vi "Fixed Number Graph Read.vi"(8 "error in":errorcluster, 9 "Data to read in":T2, 10 "Channel_Timing in":T1, 11 "Report Viewer in":refnum<class "Report Viewer.lvclass">) -> (0 "error out":errorcluster, 1 "Data to read out":T2, 2 "Channel_Timing out":T1, 3 "Report Viewer out":refnum<class "Report Viewer.lvclass">, 4 "Waveform":waveform(dbl))   [LabVIEW 2019, in "Report Viewer.lvlib" / "Report Viewer.lvclass"]
uses:
  Library/Report Viewer.lvclass
  Custom Controls/Channel_Timing.ctl
  Custom Controls/Data to Read.ctl
  Library/Report Viewer.lvclass/Report Viewer.ctl
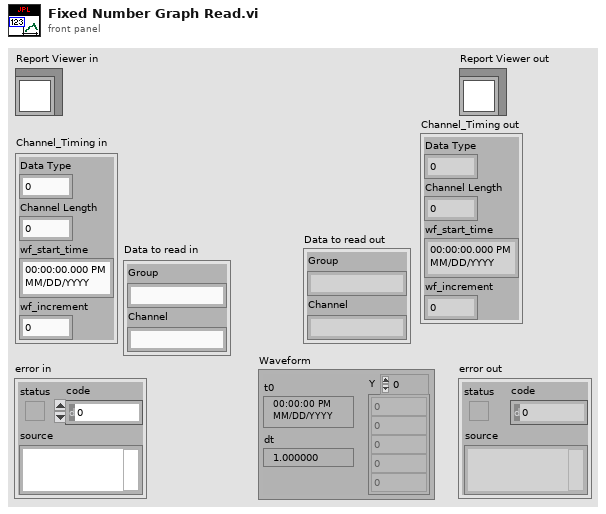
[diagram p1: front panel]
types:
  T1 = typedef "Report Viewer.lvlib/Report Viewer.lvclass/Channel_Timing.ctl" = cluster{"Data Type":u16, "Channel Length":u64, "wf_start_time":timestamp, "wf_increment":dbl}
  T2 = typedef "Report Viewer.lvlib/Report Viewer.lvclass/Data to Read.ctl" = cluster{"Group":string, "Channel":string}
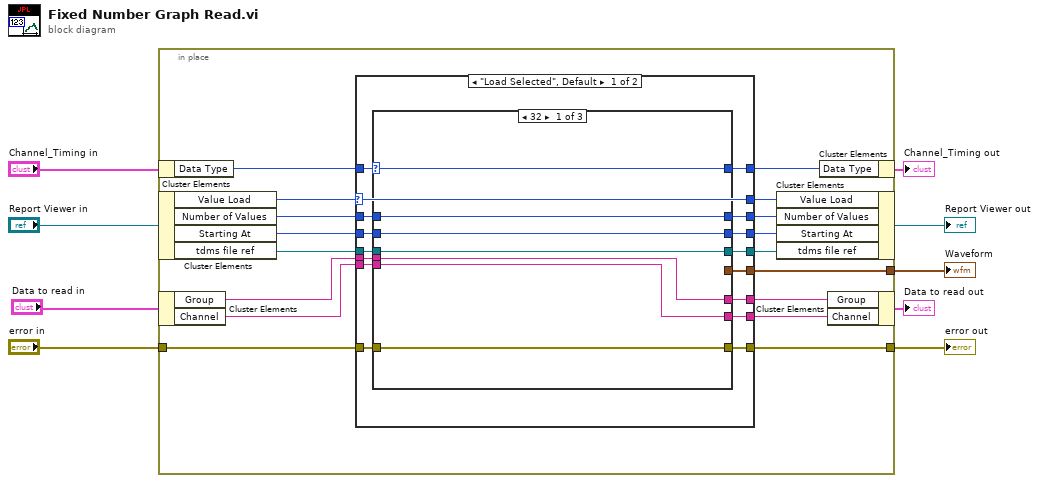
[diagram p0: block diagram]
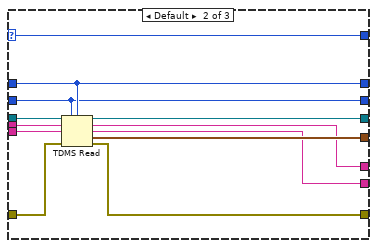
[diagram p2: hidden frame]
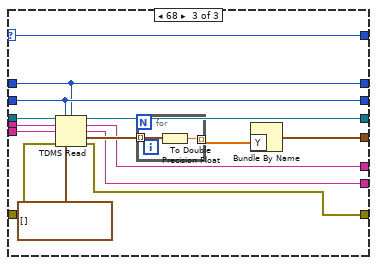
[diagram p3: hidden frame]
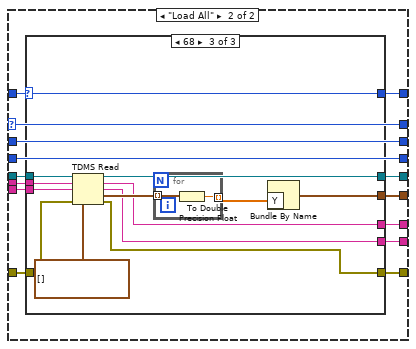
[diagram p4: hidden frame]
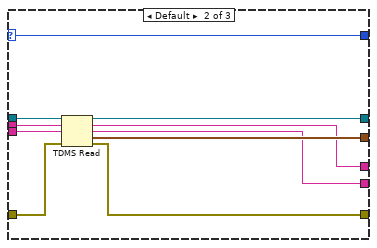
[diagram p6: hidden frame]
diagram:
  n1 = in-place {
    in-place-border: [w24] -> w7
    in-place-border: "error in" -> [w23]
    in-place-border: [w18] -> w3
    n2 = in-place-cluster #1("Channel_Timing in") -> ("Data Type"=w20:u16)
    n3 = in-place-cluster #2("Report Viewer in") -> ("Value Load"=w11:enum32{"Load All", "Load Selected"}, "Number of Values"=w21:i32, "Starting At"=w22:i32, "tdms file ref"=w26:refnum<k34>)
    n4 = in-place-cluster #3("Data to read in") -> ("Group"=w15:string, "Channel"=w14:string)
    n5 = case shown="\"Load Selected\", Default" w11 {
      selector: w11 -> [w27 w79]
      tunnel: w26 -> [w42 w92]
      tunnel: [w41 w91] -> w25
      tunnel: [w40 w90] -> w24
      tunnel: w23 -> [w39 w89]
      tunnel: w22 -> [w38 w80]
      tunnel: w21 -> [w37 w81]
      tunnel: w20 -> [w36 w88]
      tunnel: [w35 w87] -> w19
      tunnel: [w34 w86] -> w18
      tunnel: [w33 w81] -> w17
      tunnel: [w32 w80] -> w16
      tunnel: w15 -> [w31 w85]
      tunnel: w14 -> [w30 w84]
      tunnel: [w29 w83] -> w13
      tunnel: [w28 w82] -> w12
      tunnel: [w27 w79] -> w10
      frame "Load Selected", Default {
        n6 = case shown="32" w36 {
          selector: w36 -> [w49 w57 w72]
          tunnel: w42 -> [w48 w61 w76]
          tunnel: [w48 w60 w74] -> w41
          tunnel: [w45 w59 w67] -> w40
          tunnel: w39 -> [w45 w58 w75]
          tunnel: w38 -> [w46 w54 w71]
          tunnel: w37 -> [w47 w55 w70]
          tunnel: [w49 w57 w72] -> w35
          tunnel: [_ w56 w66] -> w34
          tunnel: [w47 w55 w70] -> w33
          tunnel: [w46 w54 w71] -> w32
          tunnel: w31 -> [w44 w53 w65]
          tunnel: w30 -> [w43 w52 w64]
          tunnel: [w44 w51 w63] -> w29
          tunnel: [w43 w50 w62] -> w28
          frame 32 {
          }
          frame Default {
            n7 = TDMS Read(0:w61, 1:w54, 2:w55, 5:w53, 7:w52, 11:w58) -> (4:w60:refnum<k34>, 6:w51:string, 8:w50:string, 10:w56:waveform(dbl), 15:w59:errorcluster)  [unwired: 2 in, 1 out]
          }
          frame 68 {
            n8 = TDMS Read(0:w76, 1:w71, 2:w70, 5:w65, 7:w64, 11:w75, 12:timestamp[] []) -> (4:w74:refnum<k34>, 6:w63:string, 8:w62:string, 10:w68:timestamp[], 15:w67:errorcluster)  [unwired: 1 in, 1 out]
            n9 = for {
              tunnel: w68 -> [w78] mode=indexing
              tunnel: [w77] -> w69 mode=indexing
              n10 = To Double Precision Float(number=w78) -> (double precision float=w77:dbl)
            }
            n11 = Bundle By Name("Y"=w69) -> (w66:waveform(dbl))  [unwired: 1 in]
          }
        }
      }
      frame "Load All" {
        n12 = case shown="68" w88 {
          selector: w88 -> [w97 w103 w116]
          tunnel: w92 -> [w96 w107 w120]
          tunnel: [w96 w106 w118] -> w91
          tunnel: [w95 w105 w113] -> w90
          tunnel: w89 -> [w95 w104 w119]
          tunnel: [w97 w103 w116] -> w87
          tunnel: [_ w102 w112] -> w86
          tunnel: w85 -> [w94 w101 w111]
          tunnel: w84 -> [w93 w100 w110]
          tunnel: [w94 w99 w109] -> w83
          tunnel: [w93 w98 w108] -> w82
          frame 32 {
          }
          frame Default {
            n13 = TDMS Read(0:w107, 5:w101, 7:w100, 11:w104) -> (4:w106:refnum<k34>, 6:w99:string, 8:w98:string, 10:w102:waveform(dbl), 15:w105:errorcluster)  [unwired: 4 in, 1 out]
          }
          frame 68 {
            n14 = TDMS Read(0:w120, 5:w111, 7:w110, 11:w119, 12:timestamp[] []) -> (4:w118:refnum<k34>, 6:w109:string, 8:w108:string, 10:w114:timestamp[], 15:w113:errorcluster)  [unwired: 3 in, 1 out]
            n15 = for {
              tunnel: w114 -> [w122] mode=indexing
              tunnel: [w121] -> w115 mode=indexing
              n16 = To Double Precision Float(number=w122) -> (double precision float=w121:dbl)
            }
            n17 = Bundle By Name("Y"=w115) -> (w112:waveform(dbl))  [unwired: 1 in]
          }
        }
      }
    }
    n18 = in-place-cluster #2("Value Load"=w10, "Number of Values"=w17, "Starting At"=w16, "tdms file ref"=w25) -> (→"Report Viewer out":refnum<class "Report Viewer.lvclass">)
    n19 = in-place-cluster #1("Data Type"=w19) -> (→"Channel_Timing out":T1)
    n20 = in-place-cluster #3("Group"=w13, "Channel"=w12) -> (→"Data to read out":T2)
  }
  "error out" <- w7
  "Waveform" <- w3
